vi "FlatToRichcif_channelcore_Channel.vi"(5 "OutputClusterType":T1, 11 "InputCluster":T4) -> (3 "OutputCluster":T1)   [LabVIEW 2021, in "CIF_Manager_server.lvlib"]
uses:
  CIF_Manager_server.lvlib
  cif_channelcore_Channel_Flat.ctl
  cif_channelcore_ChannelDirection.ctl
  cif_channelcore_ChannelPattern.ctl
  cif_channelcore_Channel.ctl
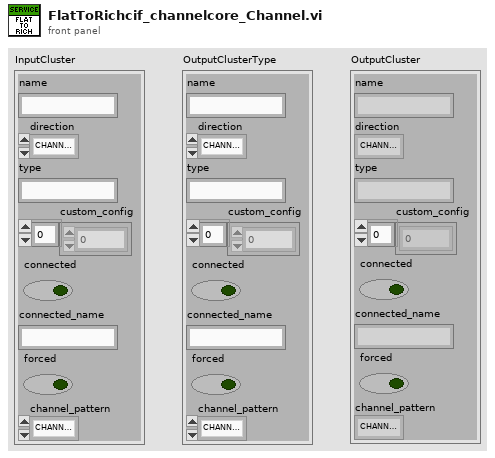
[diagram p1: front panel]
types:
  T1 = typedef "CIF_Manager_server.lvlib/cif_channelcore_Channel.ctl" = cluster{"name":string, "direction":T2, "type":string, "custom_config":u8[], "connected":bool, "connected_name":string, "forced":bool, "channel_pattern":T3}
  T2 = typedef "CIF_Manager_server.lvlib/cif_channelcore_ChannelDirection.ctl" = enum32{"CHANNELDIRECTION_UNKNOWN", "CHANNELDIRECTION_PUBLISHER", "CHANNELDIRECTION_SUBSCRIBER"}
  T3 = typedef "CIF_Manager_server.lvlib/cif_channelcore_ChannelPattern.ctl" = enum32{"CHANNELPATTERN_UNKNOWN", "CHANNELPATTERN_TAG", "CHANNELPATTERN_FIFO", "CHANNELPATTERN_MULTIFIFO", "CHANNELPATTERN_BACKPRESSUREFIFO"}
  T4 = typedef "CIF_Manager_server.lvlib/cif_channelcore_Channel_Flat.ctl" = cluster{"name":string, "direction":T2, "type":string, "custom_config":u8[], "connected":bool, "connected_name":string, "forced":bool, "channel_pattern":T3}
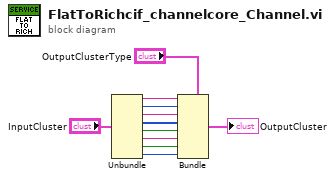
[diagram p0: block diagram]
diagram:
  n1 = Unbundle "Unbundle"("InputCluster") -> ("name"=w8:string, "direction"=w7:T2, "type"=w6:string, "custom_config"=w5:u8[], "connected"=w4:bool, "connected_name"=w3:string, "forced"=w2:bool, "channel_pattern"=w1:T3)
  n2 = Bundle "Bundle"(cluster="OutputClusterType", "name"=w8, "direction"=w7, "type"=w6, "custom_config"=w5, "connected"=w4, "connected_name"=w3, "forced"=w2, "channel_pattern"=w1) -> (→"OutputCluster":T1)
